vi "WriteTempertures.vi"() -> ()   [LabVIEW 2014]
uses:
  <userlib>/Nanonis Prog Interface V5/Nanonis Prog Interface.lvlib
panel:
  out "Temperature":dbl
  out "error out":errorcluster
  out "error":i32
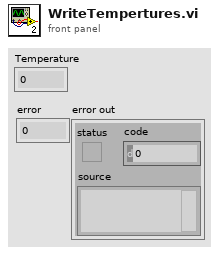
[diagram p1: front panel]
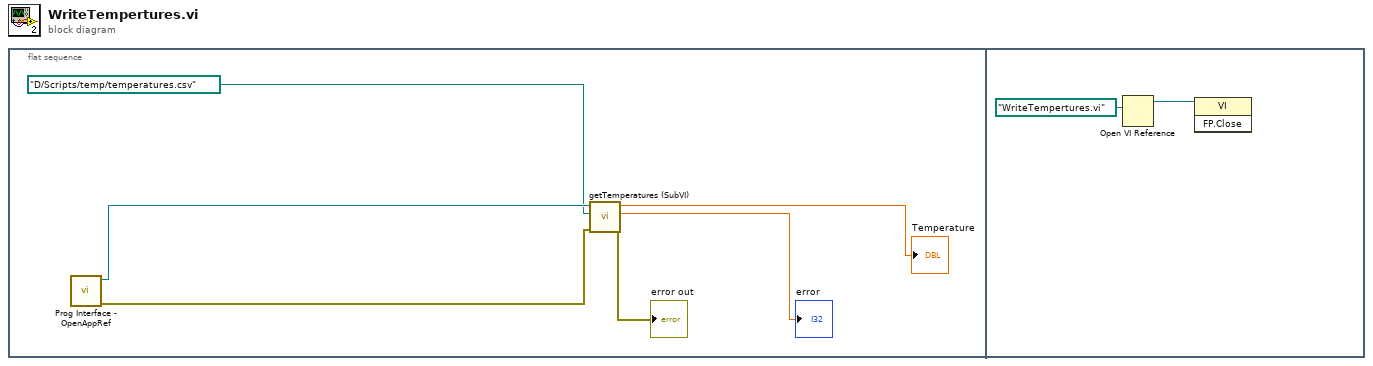
[diagram p0: block diagram]
diagram:
  n1 = flat-sequence {
    frame #0 {
      n2 = call <userlib>:"Prog Interface - OpenAppRef.vi"() -> ("Error out"=w5:errorcluster, "Application reference"=w6:refnum<vi>)  [unwired: 6 in]
      n3 = call "getTemperatures (SubVI).vi"("error in (no error)"=w5, "file path (dialog if empty)"=path "D:/Scripts/temp/temperatures.csv", "Application in"=w6) -> ("error out"=→"error out":errorcluster, "TCryo"=→"error":dbl, "TSTM"=→"Temperature":dbl)  [unwired: 5 in, 1 out]
    }
    frame #1 {
      n4 = Open VI Reference(vi path=path "WriteTempertures.vi") -> (vi reference=w7:refnum<vi>)  [unwired: 5 in, 1 out]
      n5 = invoke class="VI" method="FP.Close"(reference=w7) -> ()  [unwired: 2 in, 3 out]
    }
  }
